vi "Transcript File To DLL.vi"(4 "MinGW Path":path=path "C:/Program Files (x86)/mingw-w64/i686-8.1.0-win32-dwarf-rt_v6-rev0/mingw32/bin", 7 "dllspec alias":string="EXAMPLE_DLL", 8 "error in":errorcluster, 9 "Defines":string[](array[string])=["#define String string", "using namespace std;"], 10 "Includes":string[](array[string])=["<stdio.h>", "<string>"], 11 "vi path":path) -> (0 "error out 2":errorcluster, 1 "transcripted code":string, 2 "standard error":string, 3 "standard output":string)   [LabVIEW 2014]
panel:
  in  "Compile?":bool=TRUE
  in  "Create .h file?":bool=TRUE
  out "commands to compile DLL":string
  out "error out":errorcluster
  # "MinGW was used to build this example. This application was created based on:\nhttp://www.mingw.org/wiki/sampledll"
  # "To prove functionality create user executable \"test_example.cpp\" inside build directory:\n\n#include <stdio.h>\n#include \"example_dll.h\"\n\nint main(void)\n{\n        //LuboJ. don't forget LabVIEW transcriptor prefix for SubVIs!\n        \n        printf(\"%d\\n\", LVSubVI_Double(7));    //there is used in call generated function prefix LVSubVI_\n        LVSubVI_CppFunc();                            //there is used in call generated function prefix LVSubVI_\n\n        return 0;\n}\n\n\nCOMPILE IT USING:\ng++ -c test_example_dll.cpp\ng++ -o example_exe.exe test_example_dll.o -L. -lexample_dll\n\nRUN IT:\nexample_exe.exe"
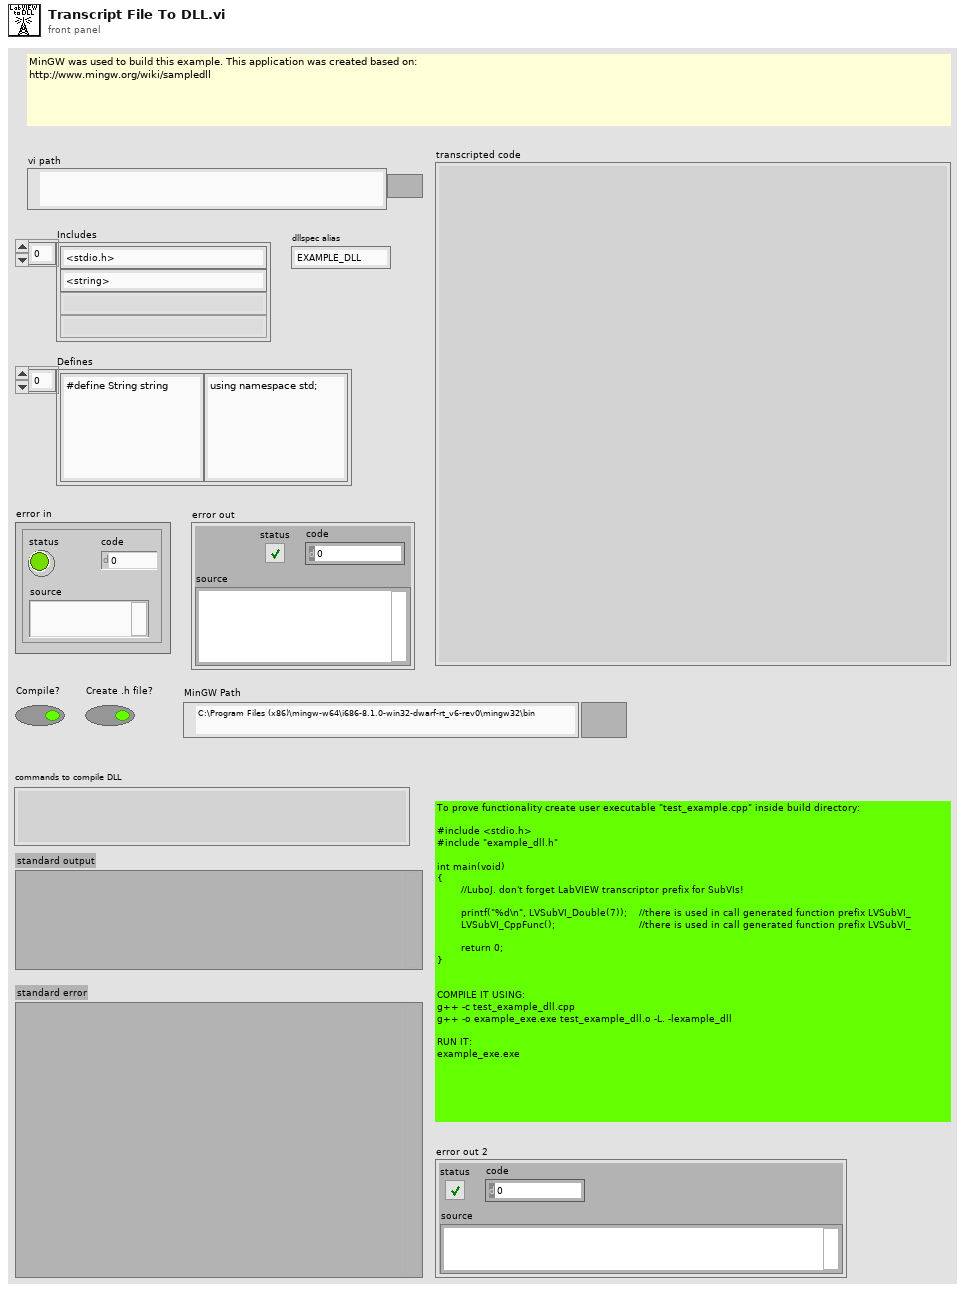
[diagram p1: front panel]
types:
  T1 = enum16{"open", "replace", "create", "open or create", "replace or create", "replace or create with confirmation"}
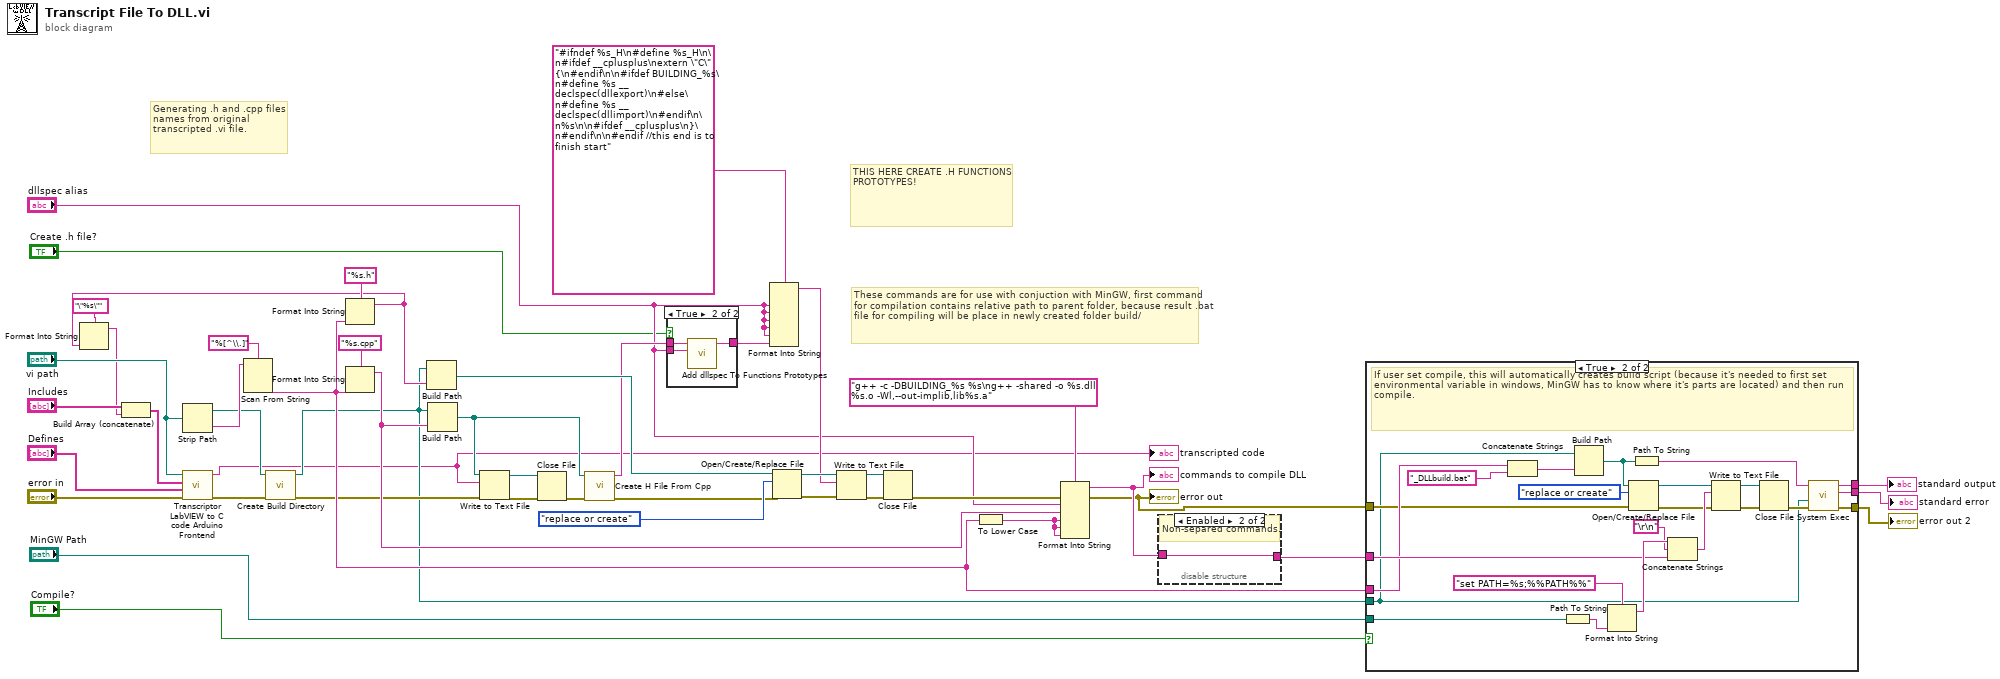
[diagram p0: block diagram]
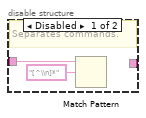
[diagram p3: hidden frame]
diagram:
  # "THIS HERE CREATE .H FUNCTIONS PROTOTYPES!"
  # "These commands are for use with conjuction with MinGW, first command for compilation contains relative path to parent folder, because result .bat file for compiling will be place in newly created folder build/"
  # "Generating .h and .cpp files names from original transcripted .vi file."
  n1 = Strip Path(path="vi path") -> (stripped path=w5:path, name=w43:string)
  n2 = Scan From String(format string="%[^\\.]", input string=w43) -> (output 1=w12:string)  [unwired: 3 in, 3 out]
  n3 = Format Into String(format string="%s.h", w12) -> (resulting string=w16:string)  [unwired: 2 in, 1 out]
  n4 = Format Into String(format string="\"%s\"", w16) -> (resulting string=w17:string)  [unwired: 2 in, 1 out]
  n5 = Build Array (concatenate)("Includes", w17) -> (w19:string[])
  n6 = call <vilib>:"Transcriptor LabVIEW to C code Arduino Frontend.vi"("error in"="error in", "Defines"="Defines", "Includes"=w19, "vi path"="vi path") -> ("error out"=w7:errorcluster, "transcripted code"=w3:string)  [unwired: 6 in]
  "transcripted code" <- w3
  n7 = call "Create Build Directory.vi"("error in"=w7, "base path"=w5) -> ("error out"=w6:errorcluster, "build path"=w4:path)  [unwired: 8 in]
  n8 = Format Into String(format string="%s.cpp", w12) -> (resulting string=w21:string)  [unwired: 2 in, 1 out]
  n9 = Build Path(base path=w4, name or relative path=w16) -> (appended path=w33:path)
  n10 = Build Path(base path=w4, name or relative path=w21) -> (appended path=w30:path)
  n11 = Write to Text File(file (use dialog)=w30, text=w3, error in=w6) -> (refnum out=w34:refnum<file>, error out=w35:errorcluster)  [unwired: 1 in, 1 out]
  n12 = Close File(refnum=w34, error in=w35) -> (error out=w32:errorcluster)  [unwired: 1 out]
  n13 = call "Create H File From Cpp.vi"("error in"=w32, "file in"=w30) -> ("error out"=w31:errorcluster, "h file content"=w27:string)  [unwired: 8 in]
  n14 = case shown="True" "Create .h file?" {
    tunnel: w27 -> [_ w50]
    tunnel: [_ w49] -> w26
    tunnel: "dllspec alias" -> [_ w48]
    frame False {
    }
    frame True {
      n15 = call "Add dllspec To Functions Prototypes.vi"("dllspec token"=w48, "input string"=w50) -> ("String"=w49:string)  [unwired: 8 in, 1 out]
    }
  }
  n16 = Format Into String(format string="#ifndef %s_H\n#define %s_H\n\n#ifdef __cplusplus\nextern \"C\" {\n#endif\n\n#ifdef BUILDING_%s\n#define %s __declspec(dllexport)\n#else\n#define %s __declspec(dllimport)\n#endif\n\n%s\n\n#ifdef __cplusplus\n}\n#endif\n\n#endif //this end is to finish start", "dllspec alias", "dllspec alias", "dllspec alias", "dllspec alias", "dllspec alias", w26) -> (resulting string=w28:string)  [unwired: 2 in, 1 out]
  n17 = Open/Create/Replace File(file path (use dialog)=w33, error in=w31, operation (0:open)=T1."replace or create") -> (refnum out=w40:refnum<file>, error out=w41:errorcluster)  [unwired: 3 in, 1 out]
  n18 = Write to Text File(file (use dialog)=w40, text=w28, error in=w41) -> (refnum out=w38:refnum<file>, error out=w39:errorcluster)  [unwired: 1 in, 1 out]
  n19 = Close File(refnum=w38, error in=w39) -> (error out=w24:errorcluster)  [unwired: 1 out]
  n20 = To Lower Case(string=w12) -> (all lower case string=w22:string)
  n21 = Format Into String(format string="g++ -c -DBUILDING_%s %s\ng++ -shared -o %s.dll %s.o -Wl,--out-implib,lib%s.a", error in=w24, "dllspec alias", w21, w22, w22, w22) -> (resulting string=w15:string, error out=w13:errorcluster)  [unwired: 1 in]
  "error out" <- w13
  "commands to compile DLL" <- w15
  n22 = disable-structure shown="Enabled" {
    disable-tunnel: w15 -> [w51 w53]
    disable-tunnel: [_ w53] -> w11
    frame Disabled {
      # "Separates commands."
      n23 = Match Pattern(string=w51, regular expression="[^\\n]*") -> ()  [unwired: 1 in, 4 out]
    }
    frame Enabled {
      # "Non-separed commands."
    }
  }
  n24 = case shown="True" "Compile?" {
    tunnel: "MinGW Path" -> [_ w77]
    tunnel: w13 -> [w54 w56]
    tunnel: w12 -> [_ w64]
    tunnel: w4 -> [_ w55]
    tunnel: w11 -> [_ w71]
    tunnel: [_ w59] -> w10
    tunnel: [_ w58] -> w9
    tunnel: [w54 w57] -> w8
    frame False {
    }
    frame True {
      # "If user set compile, this will automatically creates build script (because it's needed to first set environmental variable in windows, MinGW has to know where it's parts are located) and then run compile."
      n25 = Concatenate Strings(w64, "_DLLbuild.bat" ("string")) -> (w65:string)
      n26 = Path To String(path=w77) -> (string=w75:string)
      n27 = Build Path(base path=w55, name or relative path=w65) -> (appended path=w61:path)
      n28 = Format Into String(format string="set PATH=%s;%%PATH%%" ("command line"), w75) -> (resulting string=w73:string)  [unwired: 2 in, 1 out]
      n29 = Open/Create/Replace File(file path (use dialog)=w61, error in=w56, operation (0:open)=T1."replace or create") -> (refnum out=w68:refnum<file>, error out=w69:errorcluster)  [unwired: 3 in, 1 out]
      n30 = Path To String(path=w61) -> (string=w60:string)
      n31 = Concatenate Strings(w73, "\r\n", w71) -> (w70:string)
      n32 = Write to Text File(file (use dialog)=w68, text=w70, error in=w69) -> (refnum out=w66:refnum<file>, error out=w67:errorcluster)  [unwired: 1 in, 1 out]
      n33 = Close File(refnum=w66, error in=w67) -> (error out=w62:errorcluster)  [unwired: 1 out]
      n34 = call <vilib>:"System Exec.vi"("error in (no error)"=w62, "working directory"=w55, "command line"=w60) -> ("error out"=w57:errorcluster, "standard error"=w58:string, "standard output"=w59:string)  [unwired: 5 in, 1 out]
    }
  }
  "standard output" <- w10
  "standard error" <- w9
  "error out 2" <- w8
